vi "set position.vi"(8 "error in (no error)":errorcluster, 10 "the_set_position":T1, 11 "id":i32) -> (0 "error out":errorcluster, 3 "function return":i32)   [LabVIEW 2012, in "libximc.lvlib"]
doc: "result_t XIMC_API set_position (device_t id, const set_position_t* the_set_position);"
uses:
  libximc.lvlib
  libximc.dll
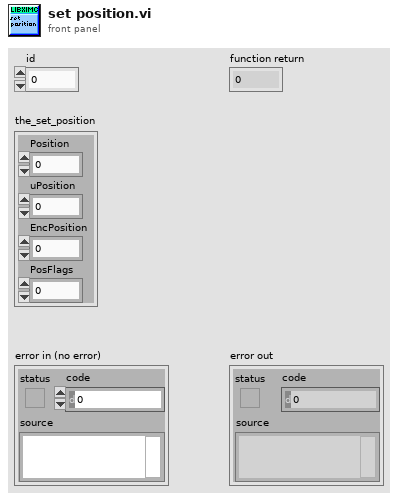
[diagram p1: front panel]
types:
  T1 = cluster{"Position":i32, "uPosition":i32, "EncPosition":i64, "PosFlags":u32}
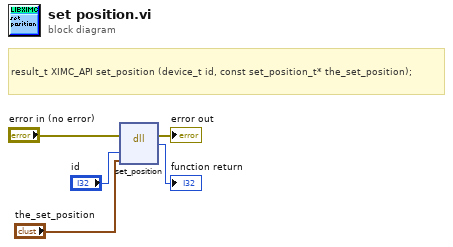
[diagram p0: block diagram]
diagram:
  # "result_t XIMC_API set_position (device_t id, const set_position_t* the_set_position);"
  n1 = dll-call lib="C:/Users/Stepan/Downloads/labview_2.9.11_testgen_thread/libximc.*" fn="set_position"(error in="error in (no error)", "id"="id", "the_set_position"="the_set_position") -> (error out=→"error out":errorcluster, →"function return":i32)  [unwired: 4 in, 1 out]
